vi "Get Control Data.vi"(8 "error in (no error)":errorcluster, 11 "TypeDef Refs":refnum<vi>[](array[refnum])) -> (0 "error out":errorcluster, 3 "Control Data":T1(array[cluster]))   [LabVIEW 2010]
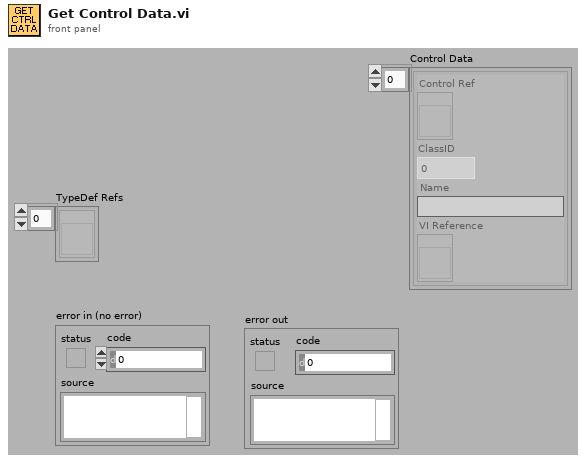
[diagram p1: front panel]
types:
  T1 = cluster{"Control Ref":refnum<vi>, "ClassID":u32, "Name":string, "VI Reference":refnum<vi>}[]
  T2 = cluster{"Control Ref":refnum<vi>, "ClassID":u32, "Name":string, "VI Reference":refnum<vi>}
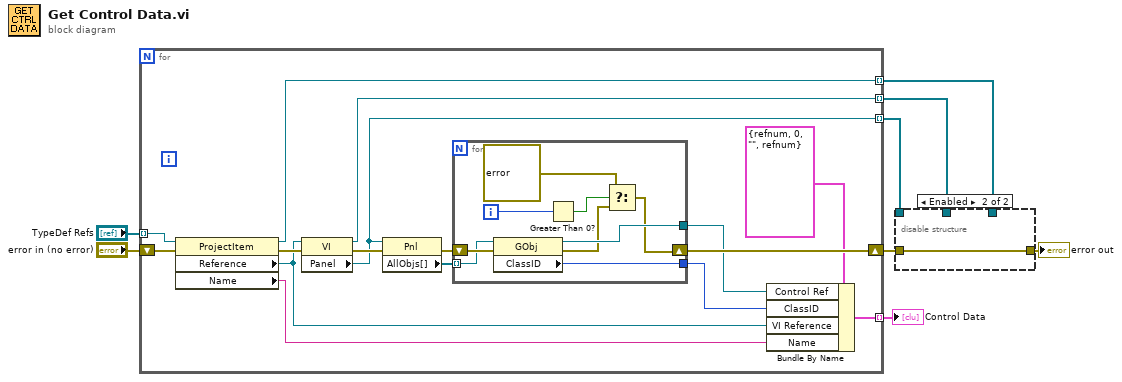
[diagram p0: block diagram]
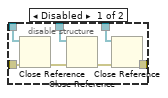
[diagram p2: hidden frame]
diagram:
  n1 = for {
    tunnel: "TypeDef Refs" -> [w24] mode=indexing
    tunnel: [w10] -> w4 mode=indexing
    tunnel: [w9] -> w5 mode=indexing
    tunnel: [w19] -> w6 mode=indexing
    shift-right: [w17] -> w7
    shift-left: "error in (no error)" -> [w18]
    tunnel: [w13] -> w1 mode=indexing
    n2 = property class="ProjectItem"(reference=w24, error in=w18) -> (reference out=w10:refnum<vi>, error out=w23:errorcluster, "Reference"=w11:refnum<vi>, "Name"=w12:string)
    n3 = property class="VI"(reference=w11, error in=w23) -> (reference out=w9:refnum<vi>, error out=w22:errorcluster, "Panel"=w19:refnum<vi>)
    n4 = property class="Pnl"(reference=w19, error in=w22) -> (error out=w21:errorcluster, "AllObjs[]"=w20:refnum<vi>[])  [unwired: 1 out]
    n5 = for {
      tunnel: w20 -> [w32] mode=indexing
      tunnel: [w31] -> w16
      shift-right: [w27] -> w17
      shift-left: w21 -> [w33]
      tunnel: [w25] -> w15
      i -> [w30]
      n6 = property class="GObj"(reference=w32, error in=w33) -> (reference out=w31:refnum<vi>, error out=w29:errorcluster, "ClassID"=w25:u32)
      n7 = Greater Than 0?(x=w30) -> (x > 0?=w28:bool)
      n8 = Select(t=errorcluster {"status"=TRUE, "code"=-88888, "source"="TypeDef contains more than 1 control.  This should never happen."}, s=w28, f=w29) -> (s? t:f=w27:errorcluster)
    }
    n9 = Bundle By Name(cluster=T2 {"Control Ref"=refnum, "ClassID"=0, "Name"="", "VI Reference"=refnum} ("output cluster"), "Control Ref"=w16, "ClassID"=w15, "VI Reference"=w11, "Name"=w12) -> (w13:T2)
  }
  "Control Data" <- w1
  n10 = disable-structure shown="Enabled" {
    disable-tunnel: [w40 w41] -> w8
    disable-tunnel: w7 -> [w38 w41]
    disable-tunnel: w6 -> [w36 _]
    disable-tunnel: w5 -> [w35 _]
    disable-tunnel: w4 -> [w34 _]
    frame Disabled {
      n11 = Close Reference(reference=w36, error in (no error)=w38) -> (error out=w39:errorcluster)
      n12 = Close Reference(reference=w35, error in (no error)=w39) -> (error out=w37:errorcluster)
      n13 = Close Reference(reference=w34, error in (no error)=w37) -> (error out=w40:errorcluster)
    }
    frame Enabled {
    }
  }
  "error out" <- w8
